vi "Modbus_ReadMeasurements.vi"(8 "error in (no error)":errorcluster, 11 "MB session in":refnum<class "MB_Master.lvclass">) -> (0 "error out":errorcluster, 1 "System \nStatus":u16, 2 "Measurements":T1, 3 "MB session out":refnum<class "MB_Master.lvclass">)   [LabVIEW 2026]
uses:
  <vilib>/Plasmionique/MB Master/MB_Master/MB_Master.lvclass
  MotorMeasurements.ctl
  <vilib>/Plasmionique/MB Master/MB Master.lvlib
panel:
  out "Vibration (mm/s)":dbl
  out "Torque (Nm)":dbl
  out "Temperature (°C)":dbl
  out "Current (A)":dbl
  out "Vibration \nRaw":u16
  out "Torque \nRaw":u16
  out "Temperature \nRaw":u16
  out "Current \nRaw":u16
  out "Actual RPM \nRaw":u16
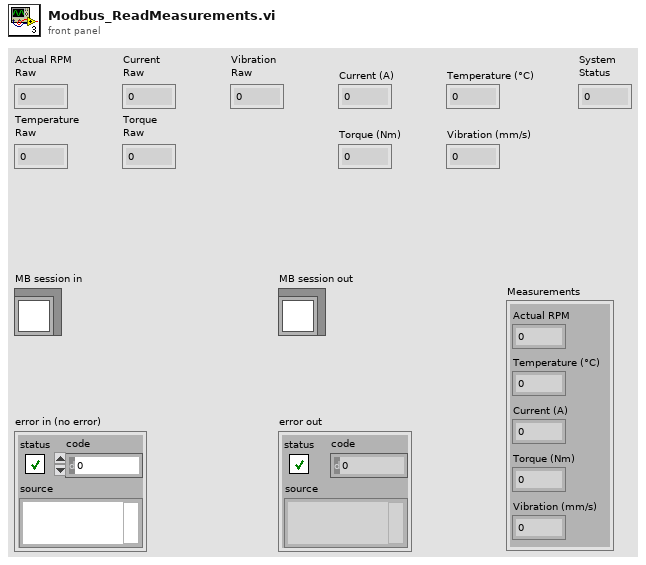
[diagram p1: front panel]
types:
  T1 = typedef "MotorMeasurements.ctl" = cluster{"Temperature (°C)":dbl, "Current (A)":dbl, "Torque (Nm)":dbl, "Vibration (mm/s)":dbl, "Actual RPM":dbl}
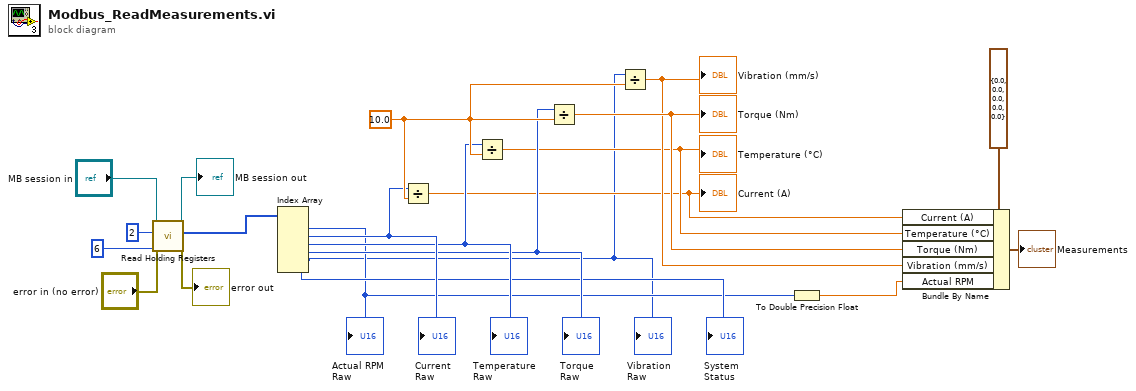
[diagram p0: block diagram]
diagram:
  w14 = 10.0
  n1 = call <vilib>:"Read Holding Registers.vi"("error in (no error)"="error in (no error)", "quantity"=u16 6, "starting address"=u16 2, "MB session in"="MB session in") -> ("error out"=→"error out":errorcluster, "Registers"=w15:u16[], "MB session out"=→"MB session out":refnum<class "MB_Master.lvclass">)  [unwired: 5 in]
  n2 = Index Array(array=w15) -> (element #1=w3:u16, element #2=w13:u16, element #3=w12:u16, element #4=w11:u16, element #5=w1:u16, element #6=→"System \nStatus":u16)  [unwired: 6 in]
  "Actual RPM \nRaw" <- w3
  "Current \nRaw" <- w13
  "Temperature \nRaw" <- w12
  "Torque \nRaw" <- w11
  "Vibration \nRaw" <- w1
  n3 = Divide(x=w13, y=w14) -> (x/y=w5:dbl)
  "Current (A)" <- w5
  n4 = Divide(x=w12, y=w14) -> (x/y=w6:dbl)
  "Temperature (°C)" <- w6
  n5 = Divide(x=w11, y=w14) -> (x/y=w8:dbl)
  "Torque (Nm)" <- w8
  n6 = Divide(x=w1, y=w14) -> (x/y=w7:dbl)
  "Vibration (mm/s)" <- w7
  n7 = To Double Precision Float(number=w3) -> (double precision float=w2:dbl)
  n8 = Bundle By Name(cluster=T1 {"Temperature (°C)"=0.0, "Current (A)"=0.0, "Torque (Nm)"=0.0, "Vibration (mm/s)"=0.0, "Actual RPM"=0.0} ("MotorMeasurements"), "Current (A)"=w5, "Temperature (°C)"=w6, "Torque (Nm)"=w8, "Vibration (mm/s)"=w7, "Actual RPM"=w2) -> (→"Measurements":T1)
